vi "Set AGC Mode.vi"(8 "error in (no error)":errorcluster, 10 "AGC Enable":bool, 11 "DeviceRefnum":u64) -> (0 "error out":errorcluster, 2 "function return":i32, 3 "DeviceRefnum Out":u64)   [LabVIEW 2014]
doc: "Enable or disable the internal digital AGC of the RTL2832."
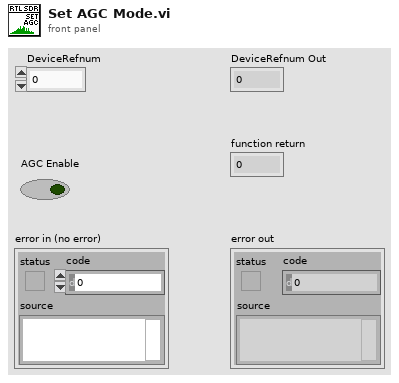
[diagram p1: front panel]
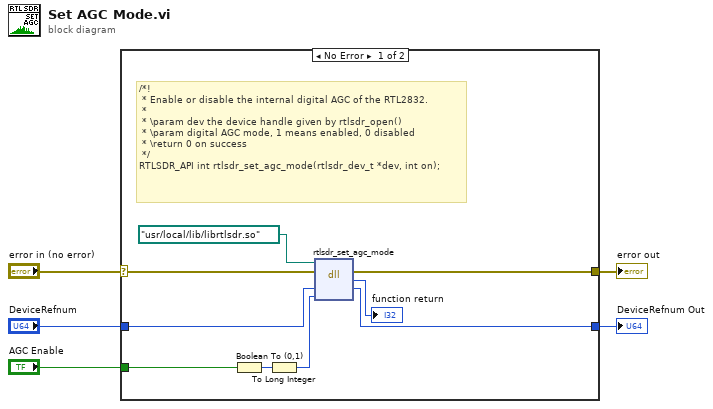
[diagram p0: block diagram]
diagram:
  n1 = case shown="No Error" "error in (no error)" {
    selector: "error in (no error)" -> [w7 w16]
    tunnel: [w13 w16] -> w5
    tunnel: "DeviceRefnum" -> [w12 w15]
    tunnel: [w11 w15] -> w3
    tunnel: "AGC Enable" -> [w10 _]
    frame No Error {
      # "/*!\n * Enable or disable the internal digital AGC of the RTL2832.\n *\n * \\param dev the device handle given by rtlsdr_open()\n * \\param digital AGC mode, 1 means enabled, 0 disabled\n * \\return 0 on success\n */\nRTLSDR_API int rtlsdr_set_agc_mode(rtlsdr_dev_t *dev, int on);"
      n2 = Boolean To (0,1)(Boolean=w10) -> (0, 1=w9:i16)
      n3 = To Long Integer(number=w9) -> (32bit integer=w8:i32)
      n4 = dll-call lib="C:/Program Files (x86)/National Instruments/LabVIEW 2016/user.lib/rtlsdr/rtlsdr.*" fn="rtlsdr_set_agc_mode"(path in=path "/usr/local/lib/librtlsdr.so", error in=w7, "DeviceRefnum"=w12, "AGC Mode"=w8) -> (error out=w13:errorcluster, "return type"=→"function return":i32, "DeviceRefnum"=w11:u64)  [unwired: 2 in, 1 out]
    }
    frame Error {
    }
  }
  "error out" <- w5
  "DeviceRefnum Out" <- w3
